vi "Save2RealTIF.vi"(3 "min_value":dbl, 4 "Specify Range?":bool=TRUE, 5 "max_value":dbl, 6 "Time Stamp?":bool=TRUE, 7 "File Name Prefix":string="ns_FLIM", 8 "error in":errorcluster, 9 "Identify Name":string="Mix_Phase0", 10 "Data 2D Array":dbl[][](array[numeric]), 11 "Parent Directory":path) -> (0 "error out":errorcluster, 2 "cancelled":bool)   [LabVIEW 2015]
uses:
  ctiff.llb/__CTIFFNewFileAndStyleFLOAT32.vi
  ctiff.llb/__CTIFFAddNewPageFLOAT32.vi
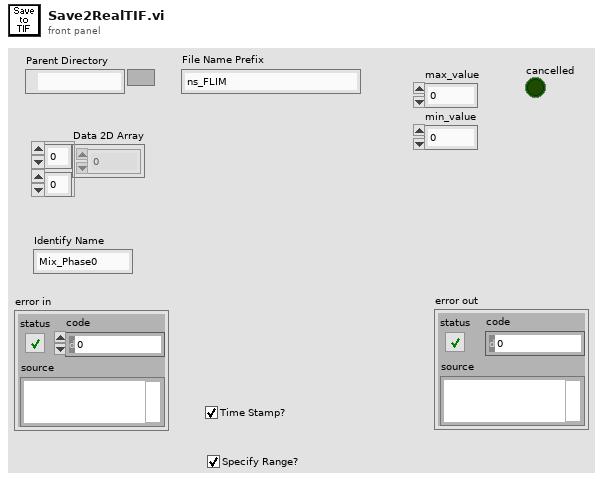
[diagram p1: front panel]
types:
  T1 = enum16{"open", "replace", "create", "open or create", "replace or create", "replace or create with confirmation"}
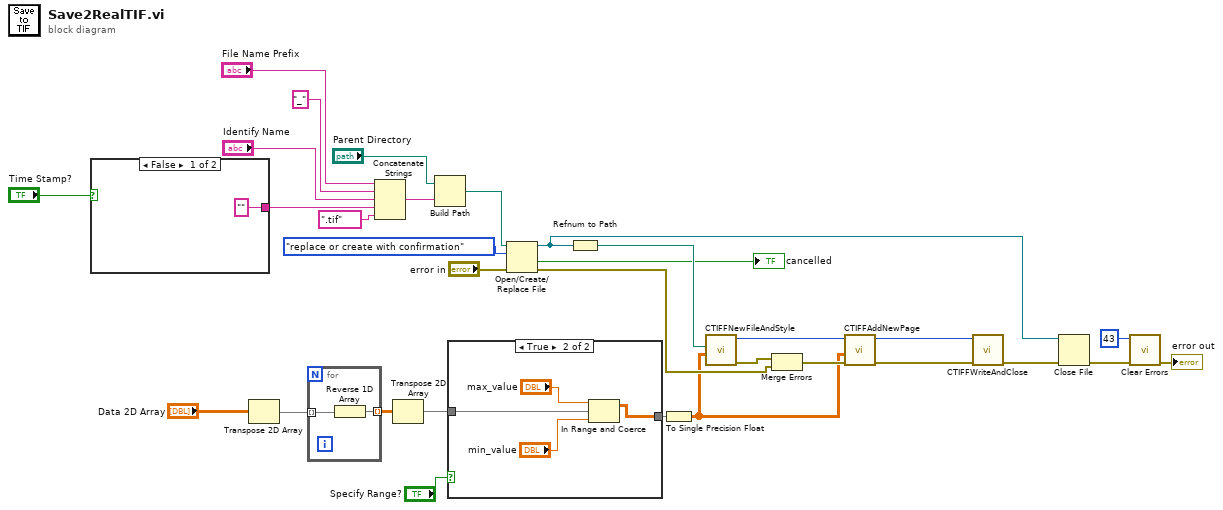
[diagram p0: block diagram]
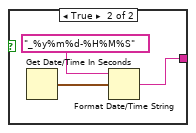
[diagram p3: hidden frame]
diagram:
  n1 = case shown="False" "Time Stamp?" {
    tunnel: ["" w33] -> w24
    frame False {
    }
    frame True {
      n2 = Get Date/Time In Seconds() -> (seconds since 1Jan1904=w34:timestamp)
      n3 = Format Date/Time String(time format string (%c)="_%y%m%d-%H%M%S", seconds (now)=w34) -> (date/time string=w33:string)  [unwired: 1 in]
    }
  }
  n4 = Transpose 2D Array(2D array="Data 2D Array") -> (transposed array=w12:dbl[][])
  n5 = for {
    tunnel: w12 -> [w37] mode=indexing
    tunnel: [w36] -> w13 mode=indexing
    n6 = Reverse 1D Array(array=w37) -> (reversed array=w36:dbl[])
  }
  n7 = Concatenate Strings("File Name Prefix", "_" ("string"), "Identify Name", w24, ".tif" ("string")) -> (w31:string)
  n8 = Transpose 2D Array(2D array=w13) -> (transposed array=w2:dbl[][])
  n9 = Build Path(base path="Parent Directory", name or relative path=w31) -> (appended path=w22:path)
  n10 = case shown="True" "Specify Range?" {
    tunnel: w2 -> [w38 w42]
    tunnel: [w38 w39] -> w1
    frame False {
    }
    frame True {
      n11 = In Range and Coerce(upper limit="max_value", x=w42, lower limit="min_value") -> (coerced(x)=w39:dbl[][])  [unwired: 1 out]
    }
  }
  n12 = Open/Create/Replace File(file path (use dialog)=w22, error in="error in", operation (0:open)=T1."replace or create with confirmation") -> (refnum out=w17:refnum<file>, cancelled=→"cancelled":bool, error out=w15:errorcluster)  [unwired: 3 in]
  n13 = Refnum to Path(1:w17) -> (0:w16:path)
  n14 = To Single Precision Float(number=w1) -> (single precision float=w3:sgl[][])
  n15 = call-poly "CTIFFNewFileAndStyle.vi"("image"=w3, "output_file"=w16) -> ("error"=w8:errorcluster, "CTIFF"=w6:i64)  [unwired: 8 in]
  n16 = Merge Errors(w8, w15) -> (w7:errorcluster)
  n17 = call-poly "CTIFFAddNewPage.vi"("error"=w7, "image"=w3, "CTIFF"=w6) -> ("error"=w4:errorcluster, "CTIFF"=w5:i64)  [unwired: 7 in]
  n18 = call "CTIFFWriteAndClose.vi"("error"=w4, "CTIFF"=w5) -> ("error"=w14:errorcluster)  [unwired: 9 in]
  n19 = Close File(refnum=w17, error in=w14) -> (error out=w18:errorcluster)  [unwired: 1 out]
  n20 = call <vilib>:"Clear Errors.vi"("error in (no error)"=w18, "specific error code to clear (0: all)"=43) -> ("error out"=→"error out":errorcluster)  [unwired: 4 in, 1 out]
